vi "Write Operation Mode.vi"(8 "error in (no error)":errorcluster, 10 "Operation Mode":T1=enum."Channel Test", 11 "rqcBob in":refnum<class "rqcBob.lvclass">) -> (0 "error out":errorcluster, 3 "rqcBob out":refnum<class "rqcBob.lvclass">)   [LabVIEW 2019, in "rqcBob.lvclass"]
uses:
  rqcBob.lvclass
  Custom Controls/rqcBob Operation Mode.ctl
  Custom Controls/rqcBob Main FPGA interface.ctl
  rqcBob.lvclass/rqcBob.ctl
  FPGA/rqcBob/Custom Controls/rqcBob Trigger Type.ctl
  <vilib>/Utility/error.llb/Error Cluster From Error Code.vi
  <vilib>/rvi/errors/niLvFpgaAdjustHostInterfaceError.vi
  <vilib>/rvi/interface/common/niFpgaWaitOnOcc.vi
  <vilib>/rvi/interface/nirviReadWriteControl/nirviReadWriteControl.xnode
  <vilib>/rvi/interface/nirviMethod/nirviMethod.xnode
  NiFpgaLv.dll
  <vilib>/rvi/interface/Simulation/niFpgaSimulationCallBeginRW.vi
  <vilib>/rvi/errors/niLvFpgaMergeErrorWithErrorCode.vi
  <vilib>/FPGAPlugInAG/Dynamic/niLvFpga_ConfigureFifo_Dynamic.vi
  <vilib>/FPGAPlugInAG/Dynamic/niLvFpga_StartFifo_Dynamic.vi
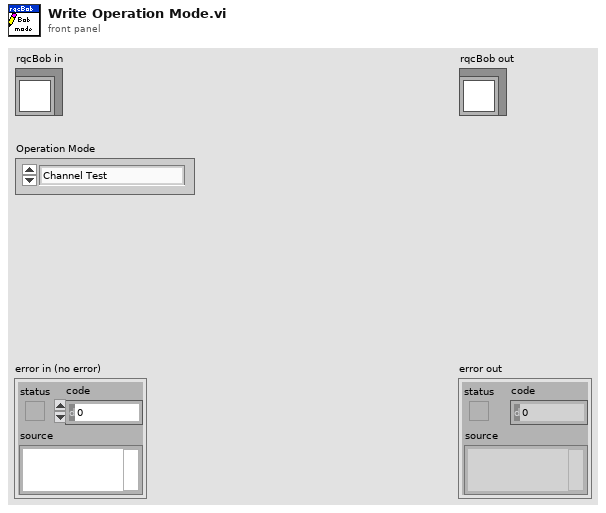
[diagram p1: front panel]
types:
  T1 = typedef "rqcBob.lvclass/rqcBob Operation Mode.ctl" = enum16{"Not Set", "Channel Test", "Key Distribution", "Modulation Level Test", "Window Test", "Delay Line Test", "Alice Modulation Level Test"}
  T2 = typedef "rqcBob.lvclass/rqcBob Main FPGA interface.ctl" = refnum<k20>
  T3 = typedef "rqcBob Trigger Type.ctl" = enum16{"software", "immediate", "DIO"}
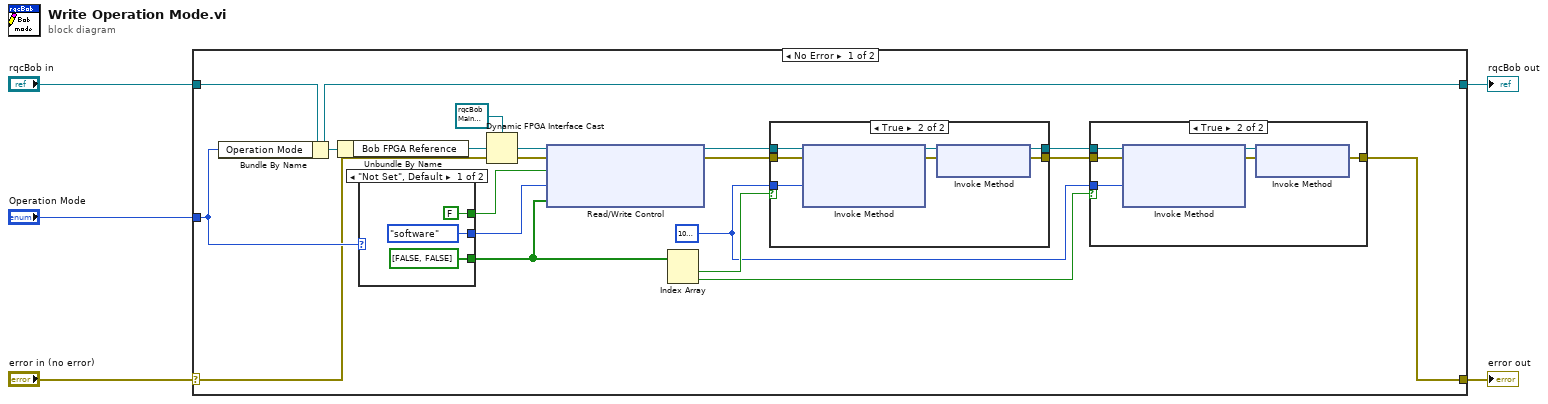
[diagram p0: block diagram]
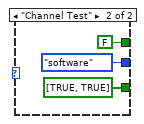
[diagram p2: hidden frame]
diagram:
  n1 = case shown="No Error" "error in (no error)" {
    selector: "error in (no error)" -> [w18 w46]
    tunnel: [w9 w46] -> w4
    tunnel: [w8 w47] -> w2
    tunnel: "rqcBob in" -> [w23 w47]
    tunnel: "Operation Mode" -> [w22 _]
    frame No Error {
      w6 = u32 1000000
      n2 = Bundle By Name(cluster=w23, "Operation Mode"=w22) -> (w8:refnum<class "rqcBob.lvclass">)
      n3 = Unbundle By Name(w8) -> ("Bob FPGA Reference"=w21:refnum<k20>)
      n4 = case shown="\"Not Set\", Default" w22 {
        tunnel: [FALSE ("PD.use window") FALSE ("PD.use window")] -> w17
        tunnel: [rqcBob_Trigger_Type."software" ("rqcBob Trigger Type") rqcBob_Trigger_Type."software" ("rqcBob Trigger Type")] -> w16
        tunnel: [bool[] [FALSE, FALSE] ("PD.detect fifo write enable") bool[] [TRUE, TRUE] ("PD.detect fifo write enable")] -> w15
        frame "Not Set", Default {
        }
        frame "Channel Test" {
        }
      }
      n5 = Dynamic FPGA Interface Cast(Session In=T2 refnum ("Bob main FPGA interface"), Type=w21) -> (Session Out=w19:T2)
      n6 = xnode "Read/Write Control"("FPGA VI Reference In"=w19, "error in"=w18, "PD.use window"=w17, "train.trigger type"=w16, "PD.detect fifo write enable"=w15) -> ("FPGA VI Reference Out"=w13:T2, "error out"=w7:errorcluster)
      n7 = Index Array(array=w15) -> (element #1=w14:bool, element #2=w12:bool)  [unwired: 2 in]
      n8 = case shown="True" w14 {
        tunnel: w13 -> [w30 w38]
        tunnel: w7 -> [w31 w37]
        tunnel: [w31 w34] -> w10
        tunnel: w6 -> [_ w33]
        tunnel: [w30 w32] -> w11
        frame False {
        }
        frame True {
          n9 = xnode "Invoke Method"("FPGA VI Reference In"=w38, "error in"=w37, "Requested Depth"=w33) -> ("FPGA VI Reference Out"=w36:T2, "error out"=w35:errorcluster)  [unwired: 1 out]
          n10 = xnode "Invoke Method"("FPGA VI Reference In"=w36, "error in"=w35) -> ("FPGA VI Reference Out"=w32:T2, "error out"=w34:errorcluster)
        }
      }
      n11 = case shown="True" w12 {
        tunnel: w11 -> [_ w45]
        tunnel: w10 -> [w39 w44]
        tunnel: [w39 w41] -> w9
        tunnel: w6 -> [_ w40]
        frame False {
        }
        frame True {
          n12 = xnode "Invoke Method"("FPGA VI Reference In"=w45, "error in"=w44, "Requested Depth"=w40) -> ("FPGA VI Reference Out"=w43:T2, "error out"=w42:errorcluster)  [unwired: 1 out]
          n13 = xnode "Invoke Method"("FPGA VI Reference In"=w43, "error in"=w42) -> ("error out"=w41:errorcluster)  [unwired: 1 out]
        }
      }
    }
    frame Error {
    }
  }
  "error out" <- w4
  "rqcBob out" <- w2
